vi "DSF.Engine.Plugin.Launch Transceiver Thread.vi"(8 "error in (no error)":errorcluster, 10 "Thread Parameters":refnum<class "Thread Parameters.lvclass">, 11 "Plugin in":refnum<class "Plugin.lvclass">) -> (0 "error out":errorcluster, 2 "Interface":refnum<class "DSF.Engine.Interface.Plugin.lvclass">, 3 "Plugin out":refnum<class "Plugin.lvclass">)   [LabVIEW 2017, in "DSF.Engine.lvlib" / "Plugin.lvclass"]
uses:
  Plugin.lvclass
  Thread Parameters/Thread Parameters.lvclass
  Interface/DSF.Engine.Interface.Plugin.lvclass
  Plugin.lvclass/Plugin.ctl
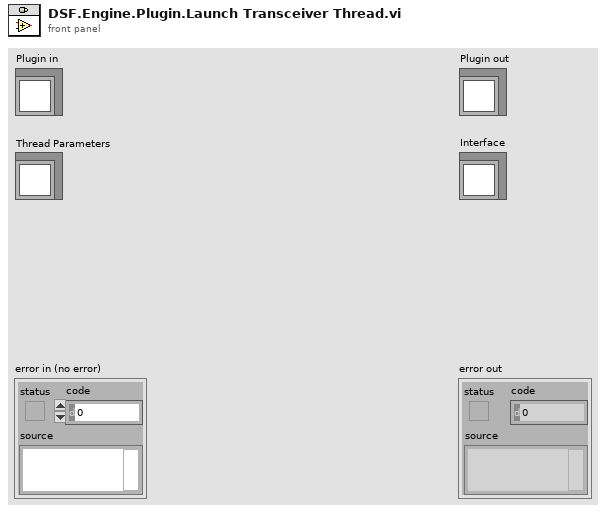
[diagram p1: front panel]
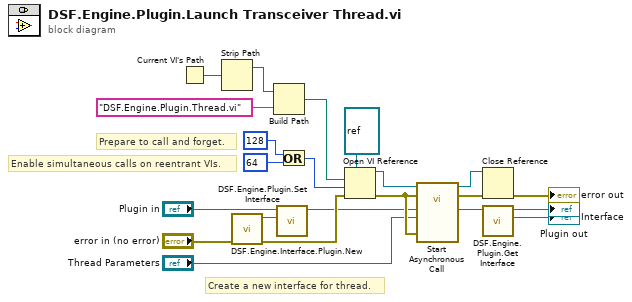
[diagram p0: block diagram]
diagram:
  # "Create a new interface for thread."
  # "Prepare to call and forget."
  # "Enable simultaneous calls on reentrant VIs."
  n1 = Current VI's Path() -> (path=w20:path)
  n2 = Strip Path(path=w20) -> (stripped path=w19:path)  [unwired: 1 out]
  n3 = call "DSF.Engine.Interface.Plugin.New.vi"("error in (no error)"="error in (no error)") -> ("error out"=w21:errorcluster, "Plugin Interface"=w4:refnum<class "DSF.Engine.Interface.Plugin.lvclass">)  [unwired: 9 in]
  n4 = Build Path(base path=w19, name or relative path="DSF.Engine.Plugin.Thread.vi") -> (appended path=w12:path)
  n5 = call "DSF.Engine.Plugin.Set Interface.vi"("Interface"=w4, "Plugin in"="Plugin in") -> ("Plugin out"=w2:refnum<class "Plugin.lvclass">)  [unwired: 9 in]
  n6 = Or(x=128 ("options"), y=64 ("options")) -> (x .or. y?=w7:i32)
  n7 = Open VI Reference(type specifier VI Refnum (for type only)=refnum<vi> refnum, vi path=w12, options=w7, error in (no error)=w21) -> (vi reference=w15:refnum<vi>, error out=w16:errorcluster)  [unwired: 2 in]
  n8 = call-by-ref "Start Asynchronous Call"(reference=w15, error in=w16, 8:"error in (no error)"=w16, "Thread Parameters"="Thread Parameters", "Plugin in"=w2) -> (reference out=w13:refnum<vi>, error out=w14:errorcluster)  [unwired: 7 in, 2 out]
  n9 = Close Reference(reference=w13, error in (no error)=w14) -> (error out=→"error out":errorcluster)
  n10 = call "DSF.Engine.Plugin.Get Interface.vi"("Plugin in"=w2) -> ("Interface"=→"Interface":refnum<class "DSF.Engine.Interface.Plugin.lvclass">, "Plugin out"=→"Plugin out":refnum<class "Plugin.lvclass">)  [unwired: 9 in]
